vi "LDO_EnviraCom_Main.vi"(1 "Vesta is working":refnum<vi>, 4 "Loop Count":refnum<vi>, 6 "State":refnum<vi>, 8 "error in":errorcluster, 9 "Retry Count":refnum<vi>, 10 "VISA resource name":refnum<visa-resource-name>="VESTA_LDO", 11 "Message Queues":T1) -> (0 "error out":errorcluster)   [LabVIEW 2023]
uses:
  Message Queue/All Message Queues.ctl
  Message Queue/Message Cluster.ctl
  Message Queue/Enqueue Message (Single).vi
  Message Queue/Message Queue.lvlib
panel:
  out "Loop Count":i32
  # "Debug"
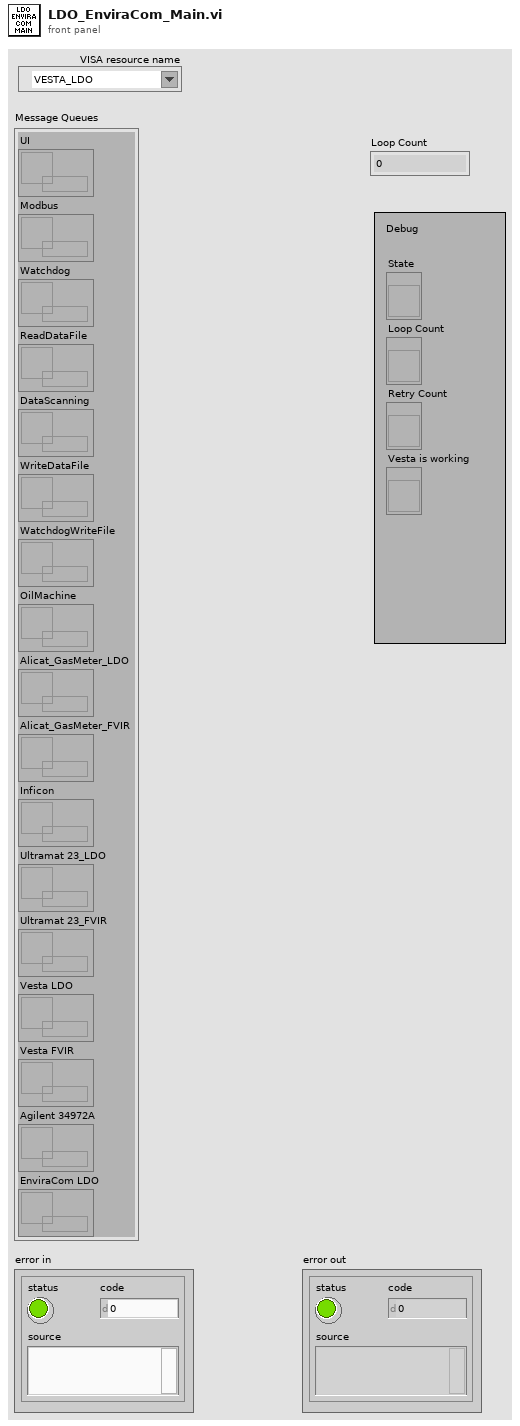
[diagram p1: front panel]
types:
  T1 = typedef "Message Queue.lvlib/All Message Queues.ctl" = cluster{"UI":refnum<queue>, "Modbus":refnum<queue>, "Watchdog":refnum<queue>, "ReadDataFile":refnum<queue>, "DataScanning":refnum<queue>, "WriteDataFile":refnum<queue>, "WatchdogWriteFile":refnum<queue>, "OilMachine":refnum<queue>, "Alicat_GasMeter_LDO":refnum<queue>, "Inficon":refnum<queue>, "Ultramat 23_LDO":refnum<queue>, "Alicat_GasMeter_FVIR":refnum<queue>, "Ultramat 23_FVIR":refnum<queue>, "Vesta LDO":refnum<queue>, "Vesta FVIR":refnum<queue>, "Agilent 34972A":refnum<queue>, "EnviraCom LDO":refnum<queue>}
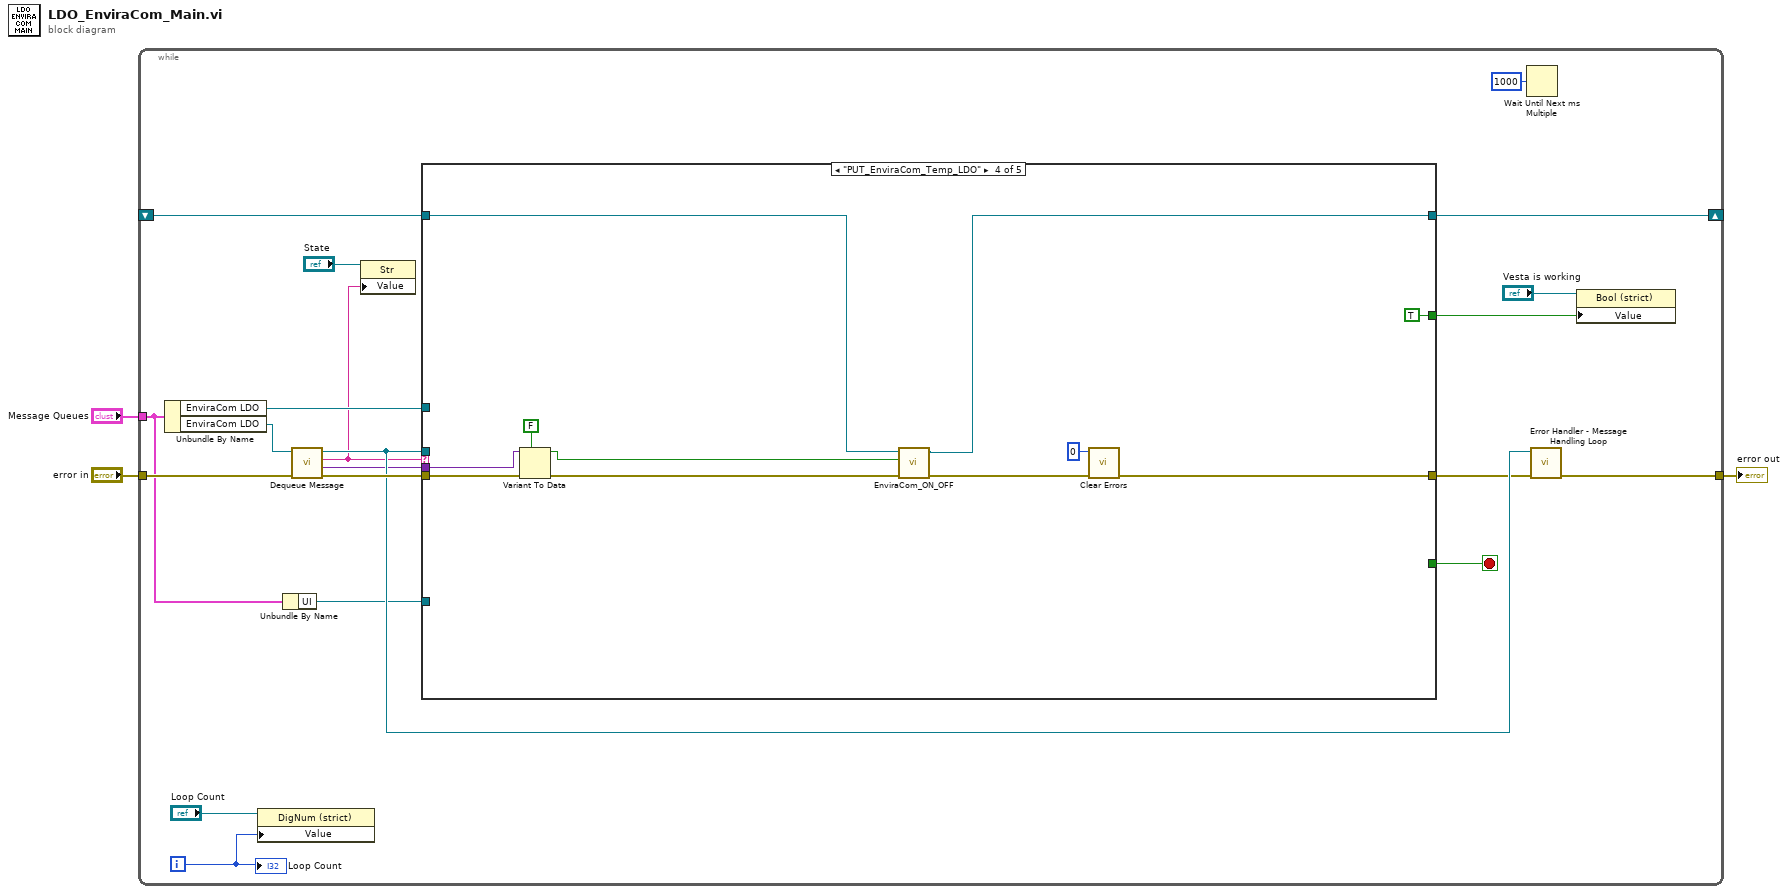
[diagram p0: block diagram]
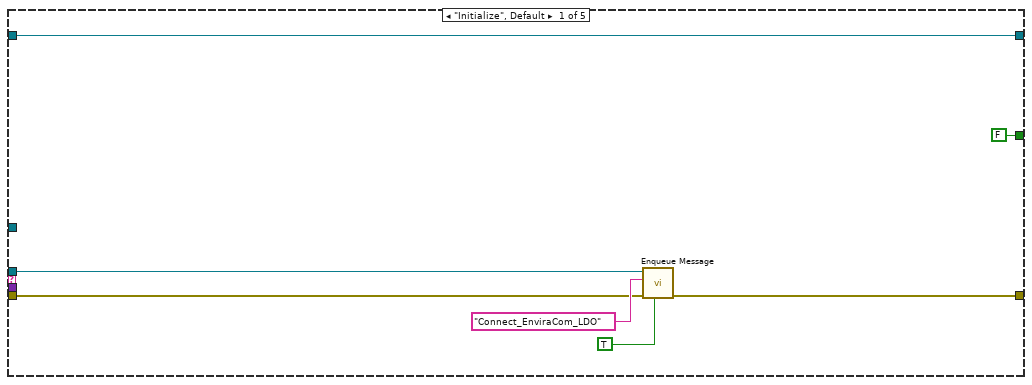
[diagram p2: hidden frame]
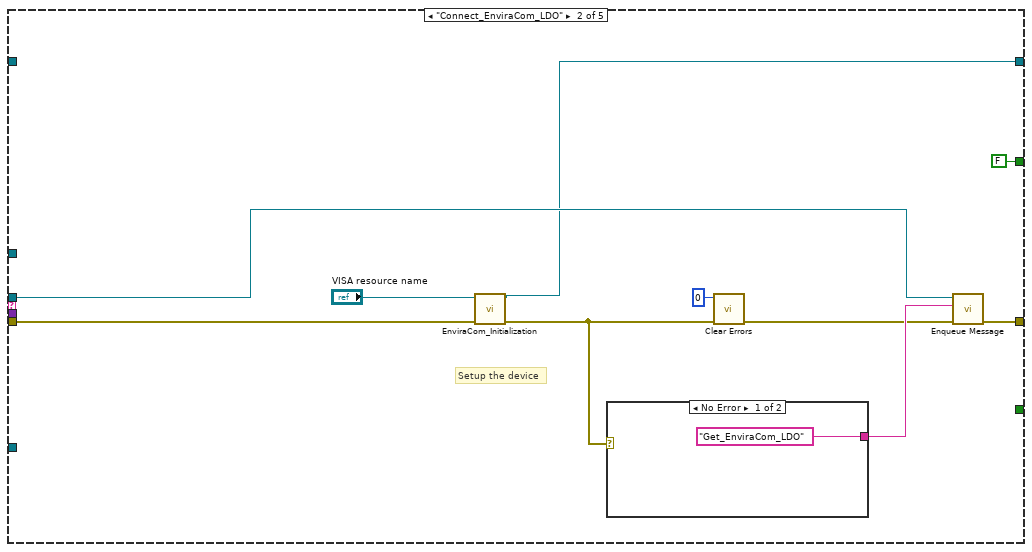
[diagram p3: hidden frame]
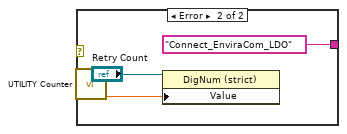
[diagram p4: hidden frame]
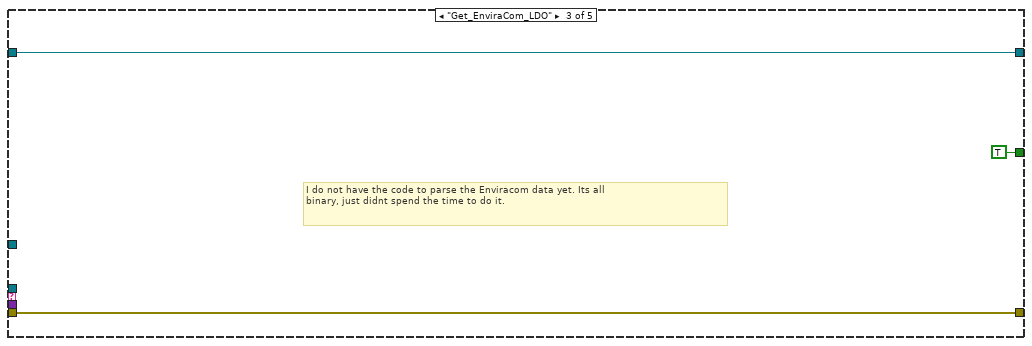
[diagram p5: hidden frame]
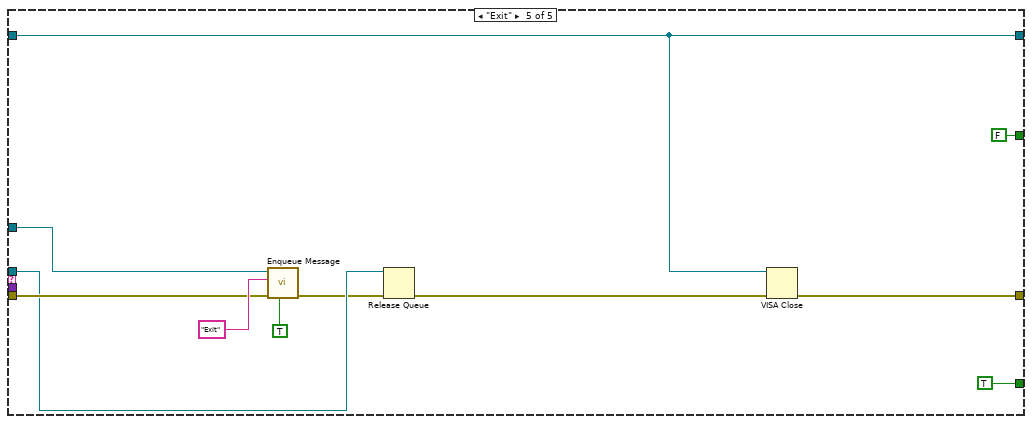
[diagram p6: hidden frame]
diagram:
  n1 = while {
    tunnel: "Message Queues" -> [w14]
    tunnel: "error in" -> [w22]
    tunnel: [w17] -> w1
    shift-right: [w12] -> _
    shift-left: _ -> [w11]
    i -> [w6]
    stop <- w20 stop-if-true
    n2 = Unbundle By Name(w14) -> ("EnviraCom LDO"=w19:refnum<queue>, "EnviraCom LDO"=w23:refnum<queue>)
    n3 = property class="DigNum (strict)"(reference="Loop Count", "Value"=w6) -> ()  [unwired: 1 in, 2 out]
    n4 = Unbundle By Name(w14) -> ("UI"=w13:refnum<queue>)
    n5 = call "Dequeue Message.vi"("error in (no error)"=w22, "Message Queue"=w23) -> ("error out"=w21:errorcluster, "Message Data"=w10:variant, "Message"=w8:string, "dup Message Queue"=w18:refnum<queue>)  [unwired: 6 in]
    n6 = property class="Str"(reference="State", "Value"=w8) -> ()  [unwired: 1 in, 2 out]
    n7 = case shown="\"PUT_EnviraCom_Temp_LDO\"" w8 {
      tunnel: w21 -> [w29 w34 w47 w58 w65]
      tunnel: [w28 w39 w47 w56 w60] -> w16
      tunnel: [_ _ _ _ TRUE] -> w20
      tunnel: w19 -> [_ _ _ _ w66]
      tunnel: w18 -> [w27 w38 _ _ w64]
      tunnel: w13 -> [_ _ _ _ _]
      tunnel: [w26 w31 w46 w50 w59] -> w12
      tunnel: w11 -> [w26 _ w46 w51 w59]
      tunnel: w10 -> [_ _ _ w57 _]
      tunnel: [FALSE ("Vesta Is Working") FALSE ("Vesta Is Working") TRUE ("Vesta Is Working") TRUE ("Vesta Is Working") FALSE ("Vesta Is Working")] -> w4
      frame "Initialize", Default {
        n8 = call-poly "Enqueue Message.vi"("Priority Message? (F)"=TRUE, "error in (no error)"=w29, "Message"="Connect_EnviraCom_LDO", "Message Queue"=w27) -> ("error out"=w28:errorcluster)  [unwired: 6 in, 1 out]
      }
      frame "Connect_EnviraCom_LDO" {
        # "Setup the device"
        n9 = call "EnviraCom_Initialization.vi"("error in (no error)"=w34, "VISA Refnum in"="VISA resource name") -> ("error out"=w33:errorcluster, "VISA Refnum out"=w31:refnum<visa-resource-name>)  [unwired: 8 in]
        n10 = case shown="No Error" w33 {
          tunnel: ["Get_EnviraCom_LDO" ("Message") "Connect_EnviraCom_LDO" ("Message")] -> w40
          frame No Error {
          }
          frame Error {
            n11 = call "UTILITY Counter.vi"() -> ("Count"=w43:dbl)  [unwired: 11 in]
            n12 = property class="DigNum (strict)"(reference="Retry Count", "Value"=w43) -> ()  [unwired: 1 in, 2 out]
          }
        }
        n13 = call <vilib>:"Clear Errors.vi"("error in (no error)"=w33, "specific error code to clear (0: all)"=0) -> ("error out"=w37:errorcluster)  [unwired: 4 in, 1 out]
        n14 = call-poly "Enqueue Message.vi"("error in (no error)"=w37, "Message"=w40, "Message Queue"=w38) -> ("error out"=w39:errorcluster)  [unwired: 7 in, 1 out]
      }
      frame "Get_EnviraCom_LDO" {
        # "I do not have the code to parse the Enviracom data yet. Its all\nbinary, just didnt spend the time to do it."
      }
      frame "PUT_EnviraCom_Temp_LDO" {
        n15 = Variant To Data(error in=w58, type=FALSE, Variant=w57) -> (data=w48:bool, error out=w53:errorcluster)
        n16 = call "EnviraCom_ON_OFF.vi"("error in (no error)"=w53, "ON (True), OFF (False)"=w48, "VISA Refnum in"=w51) -> ("error out"=w52:errorcluster, "VISA Refnum out"=w50:refnum<visa-resource-name>)  [unwired: 7 in]
        n17 = call <vilib>:"Clear Errors.vi"("error in (no error)"=w52, "specific error code to clear (0: all)"=0) -> ("error out"=w56:errorcluster)  [unwired: 4 in, 1 out]
      }
      frame "Exit" {
        n18 = call-poly "Enqueue Message.vi"("Priority Message? (F)"=TRUE, "error in (no error)"=w65, "Message"="Exit", "Message Queue"=w66) -> ("error out"=w63:errorcluster)  [unwired: 6 in, 1 out]
        n19 = Release Queue(queue=w64, error in (no error)=w63) -> (error out=w61:errorcluster)  [unwired: 1 in, 2 out]
        n20 = VISA Close(VISA resource name=w59, error in (no error)=w61) -> (error out=w60:errorcluster)
      }
    }
    n21 = Wait Until Next ms Multiple(millisecond multiple=u32 1000) -> ()  [unwired: 1 out]
    n22 = call "Error Handler - Message Handling Loop.vi"("error in (no error)"=w16, "Message Queue"=w18) -> ("dup error in"=w17:errorcluster)  [unwired: 8 in, 1 out]
    n23 = property class="Bool (strict)"(reference="Vesta is working", "Value"=w4) -> ()  [unwired: 1 in, 2 out]
    "Loop Count" <- w6
  }
  "error out" <- w1
